vi "FYP_VI_MIDI_KeyScan.vi"(1 "KeyScan":i16) -> (0 "number":u32)   [LabVIEW 2013]
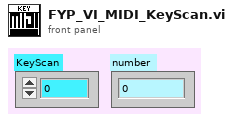
[diagram p1: front panel]
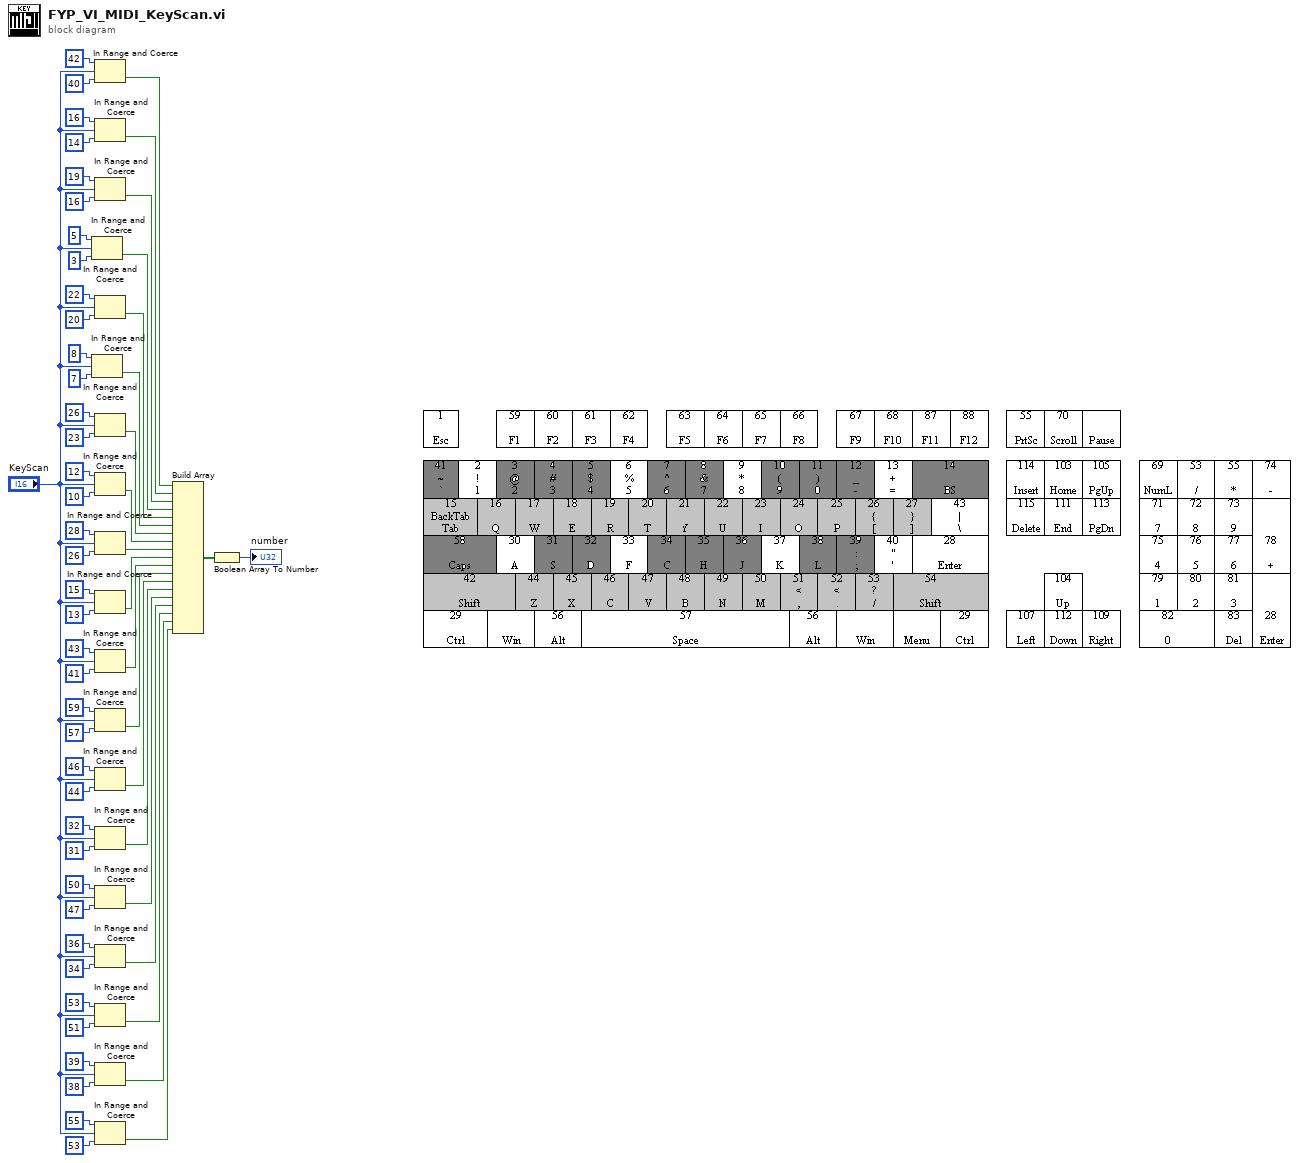
[diagram p0: block diagram]
diagram:
  n1 = In Range and Coerce(upper limit=i16 5, x="KeyScan", lower limit=i16 3) -> (In Range?=w47:bool)  [unwired: 1 out]
  n2 = In Range and Coerce(upper limit=i16 8, x="KeyScan", lower limit=i16 7) -> (In Range?=w41:bool)  [unwired: 1 out]
  n3 = In Range and Coerce(upper limit=i16 42, x="KeyScan", lower limit=i16 40) -> (In Range?=w58:bool)  [unwired: 1 out]
  n4 = In Range and Coerce(upper limit=i16 16, x="KeyScan", lower limit=i16 14) -> (In Range?=w53:bool)  [unwired: 1 out]
  n5 = In Range and Coerce(upper limit=i16 19, x="KeyScan", lower limit=i16 16) -> (In Range?=w50:bool)  [unwired: 1 out]
  n6 = In Range and Coerce(upper limit=i16 22, x="KeyScan", lower limit=i16 20) -> (In Range?=w46:bool)  [unwired: 1 out]
  n7 = In Range and Coerce(upper limit=i16 26, x="KeyScan", lower limit=i16 23) -> (In Range?=w38:bool)  [unwired: 1 out]
  n8 = In Range and Coerce(upper limit=i16 12, x="KeyScan", lower limit=i16 10) -> (In Range?=w35:bool)  [unwired: 1 out]
  n9 = In Range and Coerce(upper limit=i16 28, x="KeyScan", lower limit=i16 26) -> (In Range?=w26:bool)  [unwired: 1 out]
  n10 = In Range and Coerce(upper limit=i16 15, x="KeyScan", lower limit=i16 13) -> (In Range?=w25:bool)  [unwired: 1 out]
  n11 = In Range and Coerce(upper limit=i16 43, x="KeyScan", lower limit=i16 41) -> (In Range?=w24:bool)  [unwired: 1 out]
  n12 = In Range and Coerce(upper limit=i16 59, x="KeyScan", lower limit=i16 57) -> (In Range?=w23:bool)  [unwired: 1 out]
  n13 = In Range and Coerce(upper limit=i16 46, x="KeyScan", lower limit=i16 44) -> (In Range?=w14:bool)  [unwired: 1 out]
  n14 = In Range and Coerce(upper limit=i16 32, x="KeyScan", lower limit=i16 31) -> (In Range?=w13:bool)  [unwired: 1 out]
  n15 = In Range and Coerce(upper limit=i16 50, x="KeyScan", lower limit=i16 47) -> (In Range?=w12:bool)  [unwired: 1 out]
  n16 = In Range and Coerce(upper limit=i16 36, x="KeyScan", lower limit=i16 34) -> (In Range?=w11:bool)  [unwired: 1 out]
  n17 = In Range and Coerce(upper limit=i16 53, x="KeyScan", lower limit=i16 51) -> (In Range?=w6:bool)  [unwired: 1 out]
  n18 = In Range and Coerce(upper limit=i16 39, x="KeyScan", lower limit=i16 38) -> (In Range?=w5:bool)  [unwired: 1 out]
  n19 = In Range and Coerce(upper limit=i16 55, x="KeyScan", lower limit=i16 53) -> (In Range?=w2:bool)  [unwired: 1 out]
  n20 = Build Array(w58, w53, w50, w47, w46, w41, w38, w35, w26, w25, w24, w23, w14, w13, w12, w11, w6, w5, w2) -> (w59:bool[])
  n21 = Boolean Array To Number(Boolean array=w59) -> (number=→"number":u32)
